vi "unwrap1D.vi"(11 "Array in":dbl[][](array[numeric])) -> (3 "Array out":dbl[][](array[numeric]))   [LabVIEW 2015]
uses:
  <vilib>/Analysis/NI_AALPro.lvlib
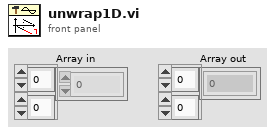
[diagram p1: front panel]
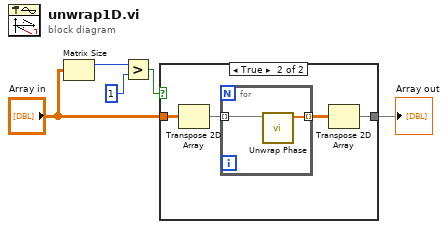
[diagram p0: block diagram]
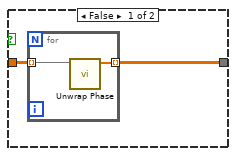
[diagram p2: hidden frame]
diagram:
  n1 = Matrix Size(0:"Array in") -> (1:w3:i32)  [unwired: 1 out]
  n2 = Greater?(x=w3, y=1) -> (0:w1:bool)
  n3 = case shown="True" w1 {
    tunnel: [w7 w13] -> w5
    tunnel: "Array in" -> [w6 w10]
    frame False {
      n4 = for {
        tunnel: [w9] -> w7 mode=indexing
        tunnel: w6 -> [w8] mode=indexing
        n5 = call <vilib>:"Unwrap Phase.vi"("Phase"=w8) -> ("Unwrapped Phase"=w9:dbl[])  [unwired: 9 in, 1 out]
      }
    }
    frame True {
      n6 = Transpose 2D Array(2D array=w10) -> (transposed array=w11:dbl[][])
      n7 = for {
        tunnel: w11 -> [w14] mode=indexing
        tunnel: [w15] -> w12 mode=indexing
        n8 = call <vilib>:"Unwrap Phase.vi"("Phase"=w14) -> ("Unwrapped Phase"=w15:dbl[])  [unwired: 9 in, 1 out]
      }
      n9 = Transpose 2D Array(2D array=w12) -> (transposed array=w13:dbl[][])
    }
  }
  "Array out" <- w5
